vi "AbortVIs.vi"   [LabVIEW 2022 SP3]
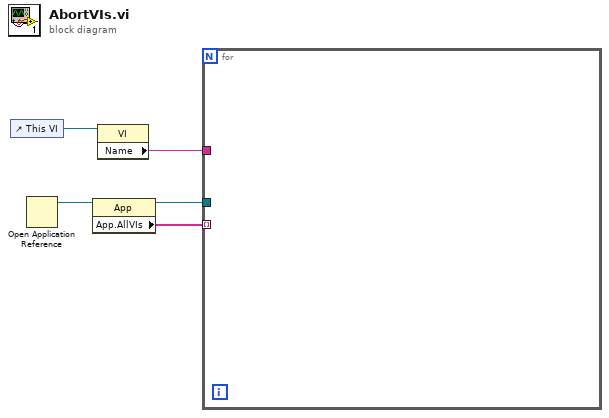
[diagram p0: block diagram]
diagram:
  n1 = control-ref of="This VI"() -> (w3:refnum<vi>)
  n2 = Open Application Reference() -> (3:w5:refnum<vi>)  [unwired: 4 in, 1 out]
  n3 = property class="App"(reference=w5) -> (reference out=w1:refnum<vi>, "App.AllVIs"=w4:string[])  [unwired: 1 in, 1 out]
  n4 = property class="VI"(reference=w3) -> ("Name"=w2:string)  [unwired: 1 in, 2 out]
  n5 = for {
    tunnel: w4 -> [_] mode=indexing
    tunnel: w2 -> [_]
    tunnel: w1 -> [_]
  }
